vi "JEN_Query.vi"(0 "System no.":i32=1 min=1 max=4 step=1, 5 "error in":errorcluster) -> (14 "Joystick control?":bool, 19 "error out":errorcluster)   [LabVIEW 2020]
doc: "Indicates whether controller joystick control is on (TRUE) or off (FALSE)."
panel:
  # "Indicates whether joystick control is on (TRUE) or off (FALSE)."
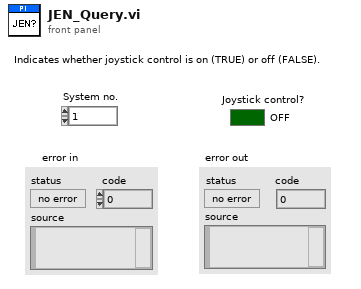
[diagram p1: front panel]
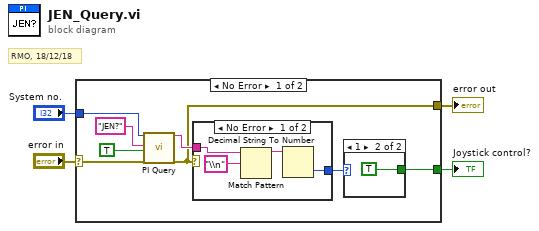
[diagram p0: block diagram]
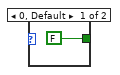
[diagram p2: hidden frame]
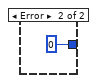
[diagram p3: hidden frame]
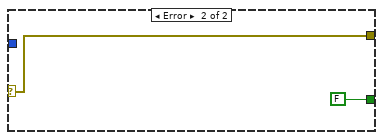
[diagram p4: hidden frame]
diagram:
  # "RMO, 18/12/18"
  n1 = case shown="No Error" "error in" {
    selector: "error in" -> [w7 w21]
    tunnel: [w5 w21] -> w4
    tunnel: "System no." -> [w11 _]
    tunnel: [w8 FALSE] -> w2
    frame No Error {
      n2 = call "PI Query.vi"("System no."=w11, "String to send"="JEN?", "Attach termination char.?"=TRUE ("Attach Linefeed?"), "error in"=w7) -> ("String read"=w6:string, "error out"=w5:errorcluster)  [unwired: 3 in, 11 out]
      n3 = case shown="No Error" w5 {
        tunnel: w6 -> [w17 _]
        tunnel: [w18 0] -> w9
        frame No Error {
          n4 = Match Pattern(string=w17, regular expression="\\n") -> (before substring=w15:string)  [unwired: 4 out]
          n5 = Decimal String To Number(string=w15) -> (number=w18:i32)  [unwired: 3 out]
        }
        frame Error {
        }
      }
      n6 = case shown="1" w9 {
        tunnel: [FALSE TRUE] -> w8
        frame 0, Default {
        }
        frame 1 {
        }
      }
    }
    frame Error {
    }
  }
  "error out" <- w4
  "Joystick control?" <- w2
